vi "sub_heading_line.vi"() -> (3 "heading_curr":cluster{dbl, dbl}[](array[cluster]))   [LabVIEW 2019]
uses:
  Ctrl/gps-databuf.ctl
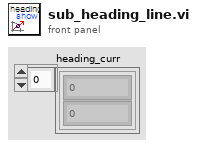
[diagram p1: front panel]
types:
  T1 = typedef "gps-databuf.ctl" = enum16{"read", "write"}
  T2 = cluster{"rawdata":string, "GPS Data":cluster{"Latitude":cluster{"Valid?":bool, "Latitude (Deg)":dbl}, "Longitude":cluster{"Valid?":bool, "Longitude (Deg)":dbl}, "Height":cluster{"Valid?":bool, "Height (m)":dbl}, "Undulation":cluster{"Valid?":bool, "Undulation(m)":dbl}, "North Vel":cluster{"Valid?":bool, "North Vel (m/s)":dbl}, "East Vel":cluster{"Valid?":bool, "East Vel (m/s)":dbl}, "Up Vel":cluster{"Valid?":bool, "Up Vel (m/s)":dbl}, "Roll":cluster{"Valid?":bool, "Roll (degrees)":dbl}, "Pitch":cluster{"Valid?":bool, "Pitch (degrees)":dbl}, "Azimuth":cluster{"Valid?":bool, "Azimuth (degrees)":dbl}, "Lat deviation":cluster{"Valid?":bool, "Lat deviation (m)":dbl}, "Long deviation":cluster{"Valid?":bool, "Long deviation (m)":dbl}, "Height deviation":cluster{"Valid?":bool, "Height deviation (m)":dbl}, "North vel deviation":cluster{"Valid?":bool, "North vel deviation (m/s)":dbl}, "East vel deviation":cluster{"Valid?":bool, "East vel deviation (m/s)":dbl}, "Up vel deviation":cluster{"Valid?":bool, "Up vel deviation (m/s)":dbl}, "Roll deviation":cluster{"Valid?":bool, "Roll deviation (degrees)":dbl}, "Pitch deviation":cluster{"Valid?":bool, "Pitch deviation (degrees)":dbl}, "Azimuth deviation":cluster{"Valid?":bool, "Azimuth deviation (degrees)":dbl}, "Ext sol status":cluster{"Valid?":bool, "Ext sol status":dbl}}, "Heading":dbl, "utm-1":cluster{"XN":dbl, "YE":dbl}}
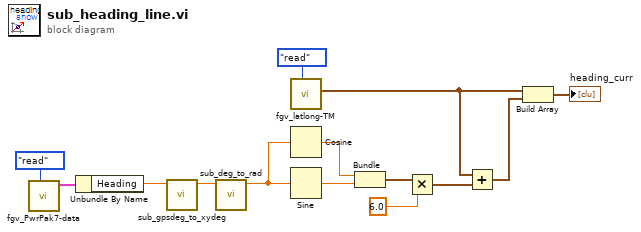
[diagram p0: block diagram]
diagram:
  n1 = call "fgv_PwrPak7-data.vi"("cmd"=gps-databuf."read") -> ("data cluster out"=w7:T2)  [unwired: 9 in, 1 out]
  n2 = Unbundle By Name(w7) -> ("Heading"=w6:dbl)
  n3 = call "sub_gpsdeg_to_xydeg.vi"("Heading"=w6) -> ("deg"=w9:dbl)  [unwired: 10 in]
  n4 = call "sub_deg_to_rad.vi"("deg in"=w9) -> ("rad out"=w10:dbl)  [unwired: 10 in]
  n5 = call "fgv_latlong-TM.vi"("cmd"=enum16{"write", "read"}."read") -> ("tm out"=w1:cluster{dbl, dbl})  [unwired: 9 in, 1 out]
  n6 = Cosine(x=w10) -> (cos(x)=w11:dbl)
  n7 = Sine(x=w10) -> (sin(x)=w12:dbl)
  n8 = Bundle(w11, w12) -> (w3:cluster{dbl, dbl})  [unwired: 1 in]
  n9 = Multiply(x=w3, y=6.0) -> (x*y=w2:cluster{dbl, dbl})
  n10 = Add(x=w1, y=w2) -> (x+y=w14:cluster{dbl, dbl})
  n11 = Build Array(w1, w14) -> (→"heading_curr":cluster{dbl, dbl}[])
